vi "Notebook Parameter Storage.vi"(6 "Get(F)/Set":bool, 7 "Notebook Parameter List":T1, 8 "Error In":errorcluster, 11 "Data in":variant) -> (0 "Error Out":errorcluster, 3 "Data out":variant)   [LabVIEW 2021, in "Notebook.lvlib"]
uses:
  Notebook.lvlib
  Notebook Parameters List.ctl
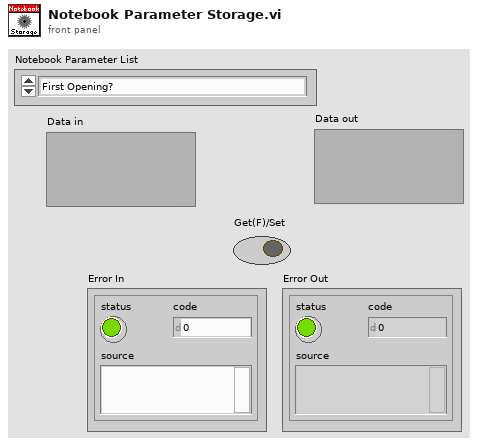
[diagram p1: front panel]
types:
  T1 = typedef "Notebook.lvlib/Notebook Parameters List.ctl" = enum16{"First Opening?", "Saved Notebook?", "Saved Notebook Path", "Beep on Error?"}
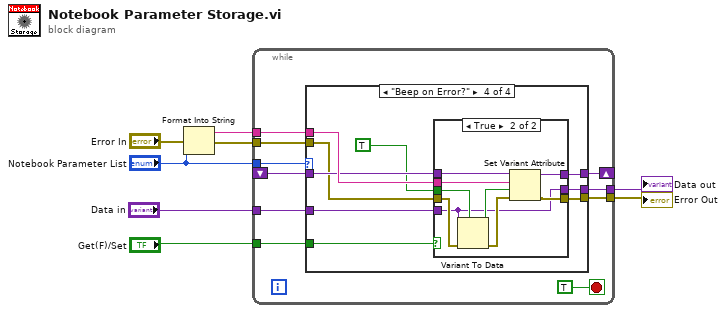
[diagram p0: block diagram]
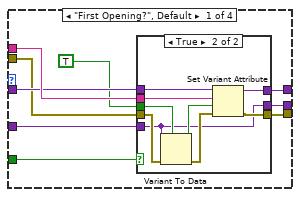
[diagram p2: hidden frame]
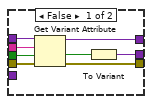
[diagram p3: hidden frame]
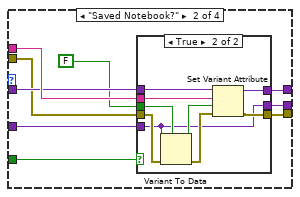
[diagram p4: hidden frame]
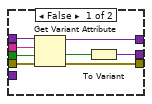
[diagram p5: hidden frame]
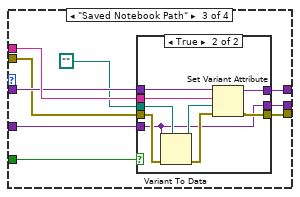
[diagram p6: hidden frame]
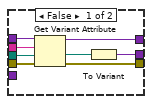
[diagram p7: hidden frame]
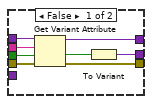
[diagram p8: hidden frame]
diagram:
  n1 = Format Into String(error in="Error In", "Notebook Parameter List") -> (resulting string=w7:string, error out=w4:errorcluster)  [unwired: 2 in]
  n2 = while {
    tunnel: "Get(F)/Set" -> [w11]
    tunnel: w7 -> [w17]
    shift-right: [w15] -> _
    shift-left: _ -> [w16]
    tunnel: "Data in" -> [w10]
    tunnel: w4 -> [w14]
    tunnel: [w13] -> w3
    tunnel: [w12] -> w2
    tunnel: "Notebook Parameter List" -> [w9]
    stop <- TRUE stop-if-true
    n3 = case shown="\"Beep on Error?\"" w9 {
      tunnel: w17 -> [w27 w53 w79 w105]
      tunnel: w16 -> [w26 w52 w78 w104]
      tunnel: [w25 w51 w77 w103] -> w15
      tunnel: w14 -> [w24 w50 w76 w102]
      tunnel: [w23 w49 w75 w101] -> w13
      tunnel: [w22 w48 w74 w100] -> w12
      tunnel: w11 -> [w21 w47 w73 w99]
      tunnel: w10 -> [w20 w46 w72 w98]
      frame "First Opening?", Default {
        n4 = case shown="True" w21 {
          tunnel: w26 -> [w35 w44]
          tunnel: w27 -> [w34 w39]
          tunnel: w24 -> [w33 w43]
          tunnel: [w32 w37] -> w23
          tunnel: [w28 w36] -> w22
          tunnel: [w30 w38] -> w25
          tunnel: TRUE -> [w29 w42]
          tunnel: w20 -> [_ w36]
          frame False {
            n5 = Get Variant Attribute(Variant=w35, name=w34, default value (empty Variant)=w29, error in=w33) -> (duplicate Variant=w30:variant, value=w31:bool, error out=w32:errorcluster)  [unwired: 1 out]
            n6 = To Variant(anything=w31) -> (Variant=w28:variant)
          }
          frame True {
            n7 = Variant To Data(error in=w43, type=w42, Variant=w36) -> (data=w41:bool, error out=w40:errorcluster)
            n8 = Set Variant Attribute(Variant=w44, name=w39, value=w41, error in=w40) -> (Variant out=w38:variant, error out=w37:errorcluster)  [unwired: 1 out]
          }
        }
      }
      frame "Saved Notebook?" {
        n9 = case shown="True" w47 {
          tunnel: w52 -> [w61 w70]
          tunnel: w53 -> [w60 w65]
          tunnel: w50 -> [w59 w69]
          tunnel: [w58 w63] -> w49
          tunnel: [w54 w62] -> w48
          tunnel: [w56 w64] -> w51
          tunnel: FALSE -> [w55 w68]
          tunnel: w46 -> [_ w62]
          frame False {
            n10 = Get Variant Attribute(Variant=w61, name=w60, default value (empty Variant)=w55, error in=w59) -> (duplicate Variant=w56:variant, value=w57:bool, error out=w58:errorcluster)  [unwired: 1 out]
            n11 = To Variant(anything=w57) -> (Variant=w54:variant)
          }
          frame True {
            n12 = Variant To Data(error in=w69, type=w68, Variant=w62) -> (data=w67:bool, error out=w66:errorcluster)
            n13 = Set Variant Attribute(Variant=w70, name=w65, value=w67, error in=w66) -> (Variant out=w64:variant, error out=w63:errorcluster)  [unwired: 1 out]
          }
        }
      }
      frame "Saved Notebook Path" {
        n14 = case shown="True" w73 {
          tunnel: w78 -> [w87 w96]
          tunnel: w79 -> [w86 w91]
          tunnel: w76 -> [w85 w95]
          tunnel: [w84 w89] -> w75
          tunnel: [w80 w88] -> w74
          tunnel: [w82 w90] -> w77
          tunnel: path "" -> [w81 w94]
          tunnel: w72 -> [_ w88]
          frame False {
            n15 = Get Variant Attribute(Variant=w87, name=w86, default value (empty Variant)=w81, error in=w85) -> (duplicate Variant=w82:variant, value=w83:path, error out=w84:errorcluster)  [unwired: 1 out]
            n16 = To Variant(anything=w83) -> (Variant=w80:variant)
          }
          frame True {
            n17 = Variant To Data(error in=w95, type=w94, Variant=w88) -> (data=w93:path, error out=w92:errorcluster)
            n18 = Set Variant Attribute(Variant=w96, name=w91, value=w93, error in=w92) -> (Variant out=w90:variant, error out=w89:errorcluster)  [unwired: 1 out]
          }
        }
      }
      frame "Beep on Error?" {
        n19 = case shown="True" w99 {
          tunnel: w104 -> [w113 w122]
          tunnel: w105 -> [w112 w117]
          tunnel: w102 -> [w111 w121]
          tunnel: [w110 w115] -> w101
          tunnel: [w106 w114] -> w100
          tunnel: [w108 w116] -> w103
          tunnel: TRUE -> [w107 w120]
          tunnel: w98 -> [_ w114]
          frame False {
            n20 = Get Variant Attribute(Variant=w113, name=w112, default value (empty Variant)=w107, error in=w111) -> (duplicate Variant=w108:variant, value=w109:bool, error out=w110:errorcluster)  [unwired: 1 out]
            n21 = To Variant(anything=w109) -> (Variant=w106:variant)
          }
          frame True {
            n22 = Variant To Data(error in=w121, type=w120, Variant=w114) -> (data=w119:bool, error out=w118:errorcluster)
            n23 = Set Variant Attribute(Variant=w122, name=w117, value=w119, error in=w118) -> (Variant out=w116:variant, error out=w115:errorcluster)  [unwired: 1 out]
          }
        }
      }
    }
  }
  "Data out" <- w2
  "Error Out" <- w3
